vi "Magnetic Sweep 1.2.vi"() -> ()   [LabVIEW 2011]
uses:
  <vilib>/Math Plots/3D Math Plots/3D Contour/3D Contour XCtrl/3D Contour.xctl
  <vilib>/Math Plots/3D Math Plots/3D Contour/3D Contour Datatype/Public/Plot Helper (Vector).vi
  <vilib>/Math Plots/3D Math Plots/3D Contour/3D Contour Datatype/3D Contour Datatype.lvclass
panel:
  out "PID command":string
  out "setpoint command":string
  out "setpoint":dbl
  out "3D Contour \n(Ramp down)":refnum<class "3D Plot Datatype.lvclass">[](xcontrol)
  out "3D Contour\n(Ramp up)":refnum<class "3D Plot Datatype.lvclass">[](xcontrol)
  in  "stop":bool
  out "error out 3":errorcluster
  out "error out 2":errorcluster
  in  "Contour plot (ramp down)":path
  in  "Raw data (ramp down)":path
  out "Elapsed Time (s)":dbl
  out "Numeric":i32
  in  "error out":errorcluster
  out "Initial Temperature":string
  out "Zero field reached":bool
  out "Target field reached":bool
  in  "Upper limite":dbl
  in  "Temperature\nramping step":dbl
  in  "Heater range":i16(ring) items=["High", "Medium", "Low"]
  in  "D gain":dbl
  in  "I gain":dbl
  in  "P gain":dbl
  in  "Contour plot (ramp up)":path
  out "Time elapsed":string
  in  "Timer":bool caption="Reset"
  in  "date format":enum16{"short", "long", "abbreviated"}(ring)
  in  "Save":bool
  in  "Raw data (ramp  up)":path
  out "Temperature vs Time":cluster{dbl[], dbl[]}(graph)
  out "current time":timestamp
  out "Magnetic\nField":cluster{dbl[], dbl[]}(graph)
  out "Current Resistance":string
  out "Current Temperature":string
  out "Current Field":string
  out "Status":string
  in  "Field Sweep":bool
  in  "Start":bool
  out "Parameter\nSetup":string
  in  "Magnetic field\nRamp rate":dbl
  in  "Traget Field":dbl
  out "Init Response":string
  in  "error in (no error)":errorcluster
  in  "IP Address":string
  in  "Ramp":bool
  in  "Update":bool
  in  "Ramp to Zero":bool
  in  "P Switch":bool
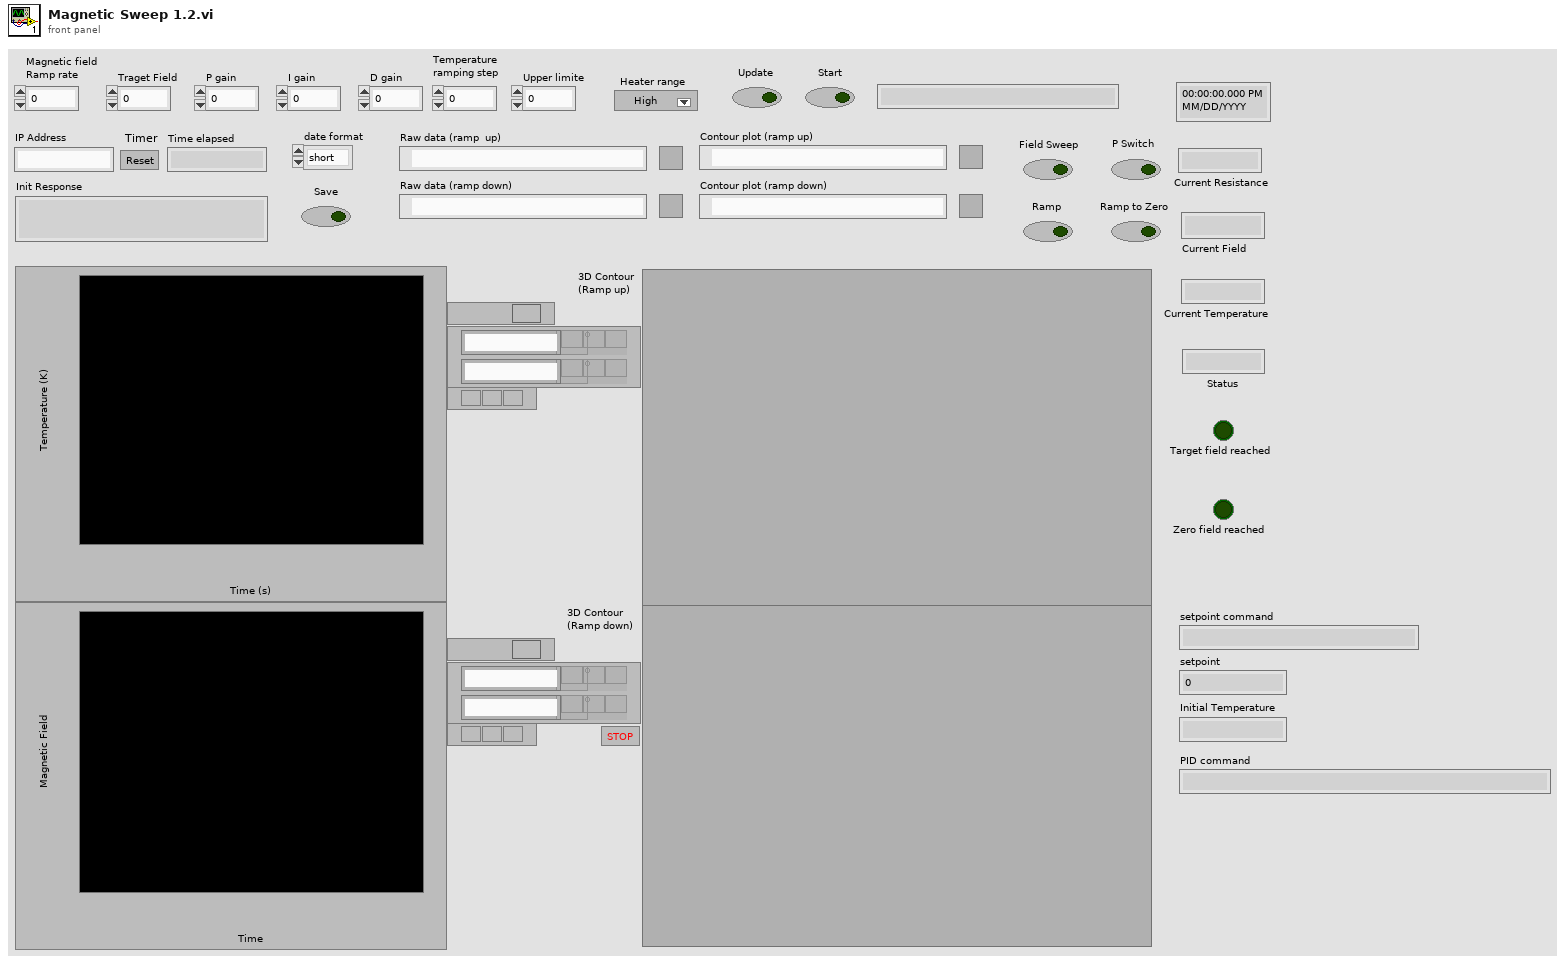
[diagram p1: front panel]
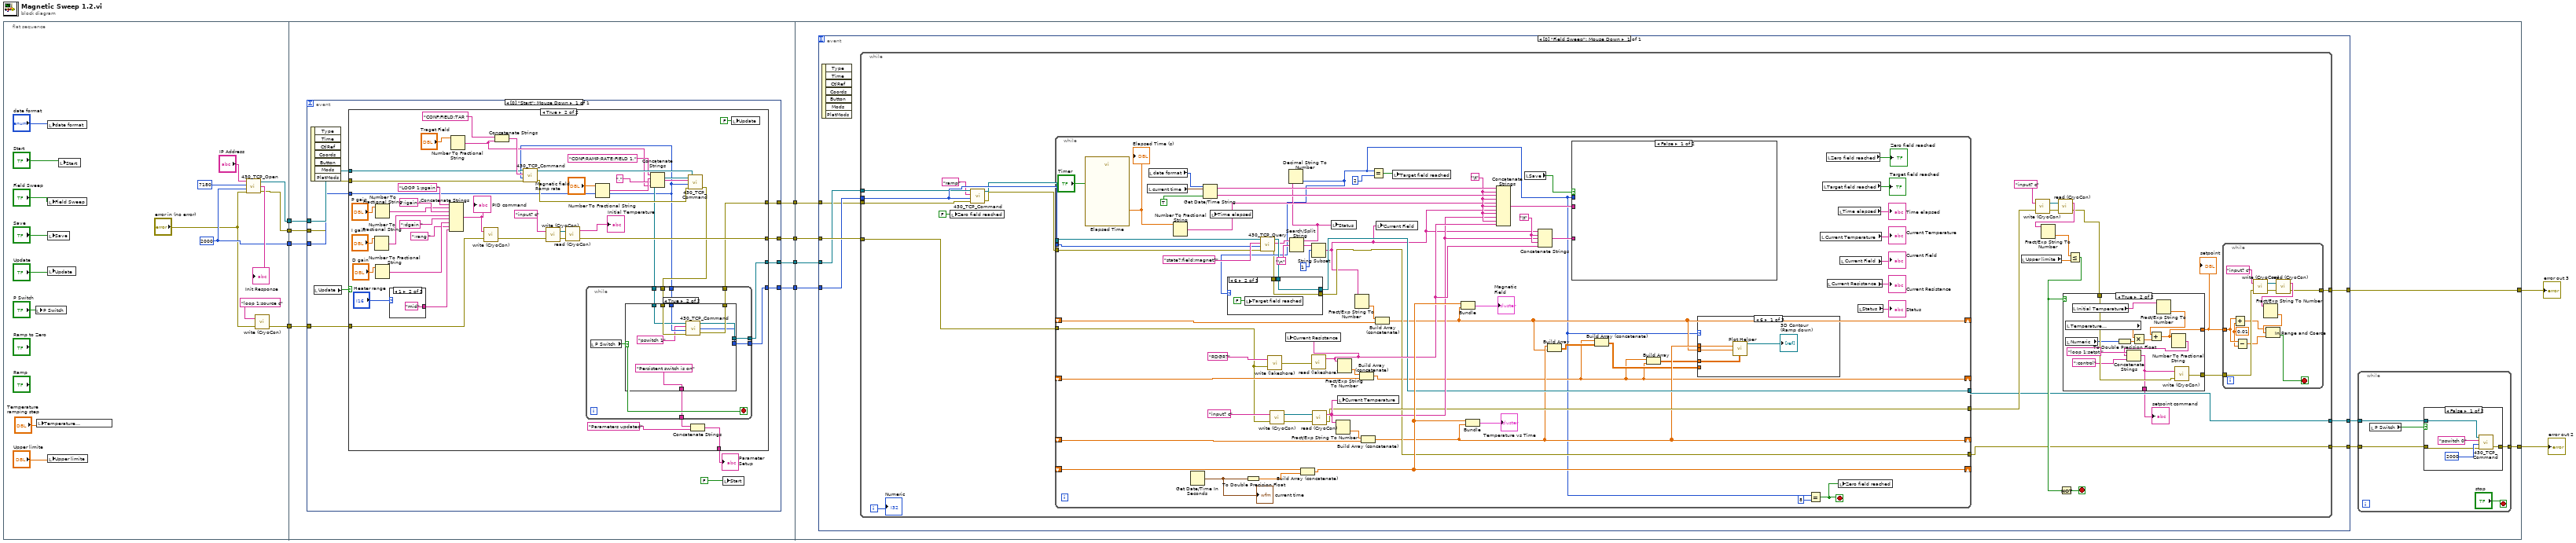
[diagram p0: block diagram]
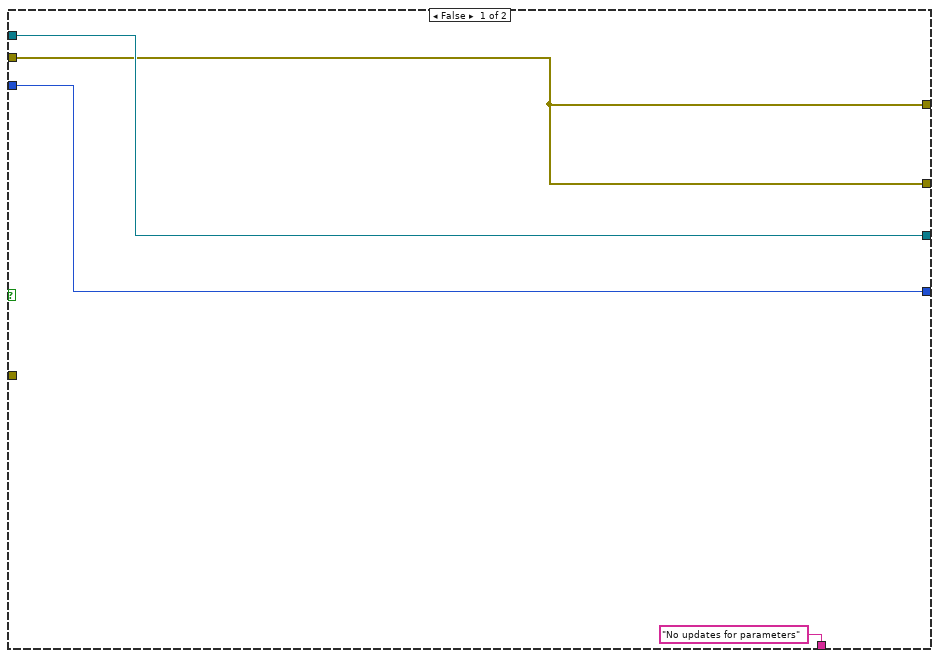
[diagram p2: hidden frame]
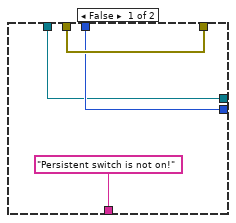
[diagram p3: hidden frame]
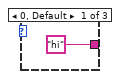
[diagram p4: hidden frame]
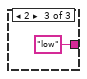
[diagram p5: hidden frame]
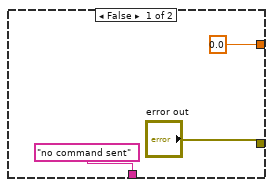
[diagram p7: hidden frame]
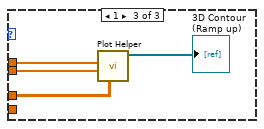
[diagram p9: hidden frame]
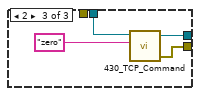
[diagram p11: hidden frame]
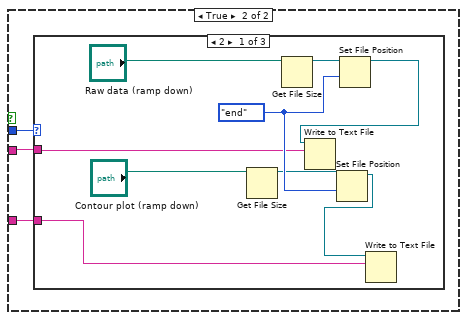
[diagram p12: hidden frame]
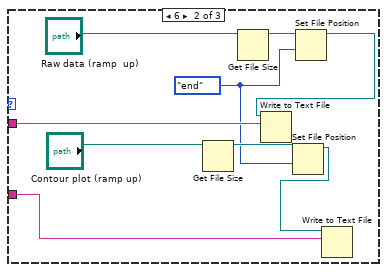
[diagram p13: hidden frame]
diagram:
  n1 = flat-sequence {
    tunnel: [w23] -> w10
    tunnel: [w22] -> w9
    tunnel: [w21] -> w8
    tunnel: [w17] -> w5
    tunnel: w10 -> [w35]
    tunnel: w9 -> [w34]
    tunnel: w8 -> [w33]
    tunnel: [w32] -> w7
    tunnel: [w31] -> w6
    tunnel: w5 -> [w30]
    tunnel: [w29] -> w4
    tunnel: [w28] -> w3
    tunnel: w7 -> [w124]
    tunnel: w6 -> [w123]
    tunnel: w4 -> [w122]
    tunnel: w3 -> [w121]
    tunnel: [w120] -> w2
    tunnel: [w118] -> w1
    frame #0 {
      w22 = 2000 ("Timeout")
      n2 = local write "P Switch"("P Switch") -> ()
      n3 = local write "Temperature\nramping step"("Temperature\nramping step") -> ()
      n4 = local write "date format"("date format") -> ()
      n5 = local write "Field Sweep"("Field Sweep") -> ()
      n6 = local write "Save"("Save") -> ()
      n7 = local write "Update"("Update") -> ()
      n8 = local write "Upper limite"("Upper limite") -> ()
      n9 = local write "Start"("Start") -> ()
      n10 = call "430_TCP_Open.vi"("IP Address"="IP Address", "TCP Port"=7180, "timeout ms (2000)"=w22, "error in (no error)"="error in (no error)") -> ("connection ID"=w23:refnum<k5>, "Init Response"=→"Init Response":string, "error out"=w21:errorcluster)  [unwired: 2 in]
      n11 = call "write (CryoCon).vi"("error in (no error)"="error in (no error)", "write buffer"="loop 1:source c") -> ("error out"=w17:errorcluster)  [unwired: 1 out]
    }
    frame #1 {
      n12 = event shown="[0] \"Start\": Mouse Down" {
        selector: _ -> [_]
        dyn-events: _ -> [_]
        timeout: _ -> [_]
        tunnel: w35 -> [w45]
        tunnel: w34 -> [w44]
        tunnel: w33 -> [w43]
        tunnel: [w42] -> w32
        tunnel: [w41] -> w31
        tunnel: w30 -> [w38]
        tunnel: [w37] -> w29
        tunnel: [w36] -> w28
        event "Start": Mouse Down {
          n13 = event-data() -> ()  [unwired: 1 in, 7 out]
          n14 = local read "Update"() -> (w46:bool)
          n15 = case shown="True" w46 {
            tunnel: w45 -> [w50 w91]
            tunnel: w44 -> [w49 w56]
            tunnel: w43 -> [w47 w80]
            tunnel: [w50 w55] -> w42
            tunnel: [w49 w54] -> w41
            tunnel: ["No updates for parameters" ("String") w51] -> w39
            tunnel: w38 -> [_ w69]
            tunnel: [w47 w61] -> w37
            tunnel: [w47 w58] -> w36
            frame False {
            }
            frame True {
              n16 = Number To Fractional String(number="I gain") -> (F-format string=w73:string)  [unwired: 3 in]
              n17 = Number To Fractional String(number="D gain") -> (F-format string=w71:string)  [unwired: 3 in]
              n18 = Number To Fractional String(number="P gain") -> (F-format string=w74:string)  [unwired: 3 in]
              n19 = case shown="1" "Heater range" {
                tunnel: ["hi" "mid" "low"] -> w66
                frame 0, Default {
                }
                frame 1 {
                }
                frame 2 {
                }
              }
              n20 = Concatenate Strings("LOOP 1:pgain " ("write buffer"), w74, ";igain " ("string"), w73, ";dgain " ("string"), w71, ";rang " ("string"), w66) -> (w70:string)
              "PID command" <- w70
              n21 = Number To Fractional String(number="Traget Field") -> (F-format string=w81:string)  [unwired: 3 in]
              n22 = call "write (CryoCon).vi"("error in (no error)"=w69, "write buffer"=w70) -> ("error out"=w62:errorcluster)  [unwired: 1 out]
              n23 = Concatenate Strings("CONF:FIELD:TAR ", w81) -> (w92:string)
              n24 = call "430_TCP_Command.vi"("error in (no error)"=w80, "Timeout"=w56, "Command"=w92, "connection ID"=w91) -> ("error out"=w90:errorcluster, "connection ID out"=w86:refnum<k5>)  [unwired: 1 out]
              n25 = call "write (CryoCon).vi"("error in (no error)"=w62, "write buffer"="input? c") -> ("error out"=w65:errorcluster, "VISA resource name out"=w64:refnum<visa-resource-name>)
              n26 = call "read (CryoCon).vi"("error in (no error)"=w65, "VISA resource name"=w64) -> ("error out"=w61:errorcluster, "read buffer"=→"Initial Temperature":string)
              n27 = Number To Fractional String(number="Magnetic field\nRamp rate") -> (F-format string=w84:string)  [unwired: 3 in]
              n28 = Concatenate Strings("CONF:RAMP:RATE:FIELD 1," ("string"), w84, "," ("string"), w81) -> (w87:string)
              n29 = call "430_TCP_Command.vi"("error in (no error)"=w90, "Timeout"=w56, "Command"=w87, "connection ID"=w86) -> ("error out"=w59:errorcluster, "connection ID out"=w57:refnum<k5>)  [unwired: 1 out]
              n30 = while {
                tunnel: w59 -> [w101]
                tunnel: [w100] -> w58
                tunnel: w57 -> [w99]
                tunnel: w56 -> [w98]
                tunnel: [w97] -> w55
                tunnel: [w96] -> w54
                tunnel: [w94] -> w52
                stop <- w95 stop-if-true
                n31 = local read "P Switch"() -> (w95:bool)
                n32 = case shown="True" w95 {
                  tunnel: w101 -> [w105 w113]
                  tunnel: [w105 w112] -> w100
                  tunnel: w99 -> [w103 w111]
                  tunnel: w98 -> [w104 w110]
                  tunnel: [w103 w109] -> w97
                  tunnel: [w104 w108] -> w96
                  tunnel: ["Persistent switch is not on!" "Persistent switch is on"] -> w94
                  frame False {
                  }
                  frame True {
                    n33 = call "430_TCP_Command.vi"("error in (no error)"=w113, "Timeout"=w110, "Command"="pswitch 1", "connection ID"=w111) -> ("error out"=w112:errorcluster, "bytes written"=w108:i32, "connection ID out"=w109:refnum<k5>)
                  }
                }
              }
              n34 = Concatenate Strings(w52, "Parameters updated" ("String")) -> (w51:string)
              n35 = local write "Update"(FALSE ("Update")) -> ()
            }
          }
          "Parameter\nSetup" <- w39
          n36 = local write "Start"(FALSE ("Set Parameter")) -> ()
        }
      }
    }
    frame #2 {
      n37 = event shown="[0] \"Field Sweep\": Mouse Down" {
        selector: _ -> [_]
        dyn-events: _ -> [_]
        timeout: _ -> [_]
        tunnel: w124 -> [w141]
        tunnel: w123 -> [w140]
        tunnel: w122 -> [w142]
        tunnel: w121 -> [w139]
        tunnel: [w138] -> w120
        tunnel: [w137] -> w119
        tunnel: [w136] -> w117
        event "Field Sweep": Mouse Down {
          n38 = event-data() -> ()  [unwired: 1 in, 7 out]
          n39 = while {
            tunnel: w142 -> [w162]
            tunnel: w140 -> [w166]
            tunnel: w141 -> [w165]
            tunnel: w139 -> [w163]
            tunnel: [w146] -> w138
            tunnel: [w145] -> w137
            tunnel: [w144] -> w136
            i -> [w159]
            stop <- w148 stop-if-true
            n40 = local write "Zero field reached"(FALSE ("Zero field reached")) -> ()
            n41 = call "430_TCP_Command.vi"("error in (no error)"=w163, "Timeout"=w166, "Command"="ramp", "connection ID"=w165) -> ("error out"=w167:errorcluster, "connection ID out"=w164:refnum<k5>)  [unwired: 1 out]
            n42 = while {
              shift-right: [w201] -> _
              shift-left: _ -> [w252]
              shift-right: [w202] -> _
              shift-left: _ -> [w257]
              shift-right: [w198] -> _
              shift-left: _ -> [w254]
              shift-right: [w247] -> _
              shift-left: _ -> [w248]
              tunnel: w167 -> [w236]
              tunnel: w166 -> [w213]
              tunnel: w164 -> [w235]
              tunnel: w162 -> [w229]
              tunnel: [w223] -> w149
              tunnel: [w211] -> w145
              tunnel: [w210] -> w144
              stop <- w215 stop-if-true
              w240 = "\t"
              w241 = "\t"
              n43 = call "Elapsed Time"("Reset"="Timer") -> ("Elapsed Time (s)"=w227:dbl)  [unwired: 11 in, 7 out]
              "Elapsed Time (s)" <- w227
              n44 = local read "current time"() -> (w238:timestamp)
              n45 = local read "date format"() -> (w230:enum16{"short", "long", "abbreviated"})
              n46 = Number To Fractional String(number=w227) -> (F-format string=w233:string)  [unwired: 3 in]
              n47 = Get Date/Time In Seconds() -> (seconds since 1Jan1904=w226:timestamp)
              "current time" <- w226
              n48 = Get Date/Time String(date format (0)=w230, seconds (now)=w238, want seconds? (F)=TRUE) -> (date string=w243:string, time string=w242:string)
              n49 = local write "Time elapsed"(w233) -> ()
              n50 = To Double Precision Float(number=w226) -> (double precision float=w249:dbl)
              n51 = call "430_TCP_Query.vi"("error in (no error)"=w236, "Timeout"=w213, "Command"="state?;field:magnet?", "connection ID"=w235) -> ("error out"=w196:errorcluster, "Response"=w209:string, "connection ID out"=w214:refnum<k5>)  [unwired: 3 in, 2 out]
              n52 = call "write (lakeshore).vi"("error in (no error)"=w229, "write buffer"="RDGR?") -> ("error out"=w256:errorcluster)
              n53 = call "write (CryoCon).vi"("error in (no error)"=w229, "write buffer"="input? c") -> ("error out"=w258:errorcluster, "VISA resource name out"=w259:refnum<visa-resource-name>)
              n54 = Search/Split String(string=w209, search string/char (-)="\n") -> (substring before match=w208:string, match + rest of string=w207:string)  [unwired: 1 in, 1 out]
              n55 = Decimal String To Number(string=w208) -> (number=w197:i32)  [unwired: 2 in, 1 out]
              n56 = case shown="6" w197 {
                tunnel: [w270 w272 w277] -> w210
                tunnel: w214 -> [w271 w274 w276]
                tunnel: [w271 w274 w275] -> w211
                tunnel: w196 -> [w270 w272 _]
                frame 0, Default {
                }
                frame 6 {
                  n57 = local write "Target field reached"(FALSE ("Target field reached")) -> ()
                }
                frame 2 {
                  n58 = call "430_TCP_Command.vi"("Command"="zero", "connection ID"=w276) -> ("error out"=w277:errorcluster, "connection ID out"=w275:refnum<k5>)  [unwired: 2 in, 1 out]
                }
              }
              n59 = Build Array (concatenate)(w248, w249) -> (w247:dbl[])
              n60 = call "read (lakeshore).vi"("error in (no error)"=w256) -> ("read buffer"=w232:string)  [unwired: 1 out]
              n61 = local write "Current Resistance"(w232) -> ()
              n62 = String Subset(string=w207, offset (0)=1) -> (substring=w205:string)  [unwired: 1 in]
              n63 = call "read (CryoCon).vi"("error in (no error)"=w258, "VISA resource name"=w259) -> ("error out"=w223:errorcluster, "read buffer"=w231:string)
              n64 = local write "Status"(w208) -> ()
              n65 = Fract/Exp String To Number(string=w231) -> (number=w251:dbl)  [unwired: 3 in, 1 out]
              n66 = Fract/Exp String To Number(string=w232) -> (number=w250:dbl)  [unwired: 3 in, 1 out]
              n67 = local write "Current Temperature"(w231) -> ()
              n68 = Fract/Exp String To Number(string=w205) -> (number=w253:dbl)  [unwired: 3 in, 1 out]
              n69 = Build Array (concatenate)(w250, w254) -> (w198:dbl[])
              n70 = Build Array (concatenate)(w251, w257) -> (w202:dbl[])
              n71 = Equal?(x=w197, y=2) -> (x = y?=w234:bool)
              n72 = Build Array (concatenate)(w253, w252) -> (w201:dbl[])
              n73 = local write "Current Field"(w205) -> ()
              n74 = local write "Target field reached"(w234) -> ()
              n75 = Bundle(w247, w201) -> (→"Magnetic\nField":cluster{dbl[], dbl[]})  [unwired: 1 in]
              n76 = Bundle(w247, w202) -> (→"Temperature vs Time":cluster{dbl[], dbl[]})  [unwired: 1 in]
              n77 = Concatenate Strings(w243, w241, w242, w241, w233, w241, w205, w241, w231, w241, w232) -> (w246:string)
              n78 = local read "Save"() -> (w225:bool)
              n79 = Concatenate Strings(w205, w240, w231, w240, w232) -> (w239:string)
              n80 = Build Array(w202, w201) -> (w212:dbl[][])
              n81 = case shown="False" w225 {
                tunnel: w246 -> [_ w281]
                tunnel: w239 -> [_ w280]
                tunnel: w197 -> [_ w279]
                frame False {
                }
                frame True {
                  n82 = case shown="2" w279 {
                    tunnel: w281 -> [w283 w299 _]
                    tunnel: w280 -> [w282 w293 _]
                    frame 2 {
                      w289 = enum16{"start", "end", "current"}."end" ("from (0:start)")
                      n83 = Get File Size(file="Contour plot (ramp down)") -> (refnum out=w288:refnum<file>)  [unwired: 1 in, 2 out]
                      n84 = Get File Size(file="Raw data (ramp down)") -> (refnum out=w285:refnum<file>)  [unwired: 1 in, 2 out]
                      n85 = Set File Position(refnum=w288, from (0:start)=w289) -> (refnum out=w290:refnum<file>)  [unwired: 2 in, 1 out]
                      n86 = Set File Position(refnum=w285, from (0:start)=w289) -> (refnum out=w286:refnum<file>)  [unwired: 2 in, 1 out]
                      n87 = Write to Text File(file (use dialog)=w286, text=w283) -> ()  [unwired: 2 in, 3 out]
                      n88 = Write to Text File(file (use dialog)=w290, text=w282) -> ()  [unwired: 2 in, 3 out]
                    }
                    frame 6 {
                      w292 = enum16{"start", "end", "current"}."end" ("from (0:start)")
                      n89 = Get File Size(file="Contour plot (ramp up)") -> (refnum out=w294:refnum<file>)  [unwired: 1 in, 2 out]
                      n90 = Get File Size(file="Raw data (ramp  up)") -> (refnum out=w297:refnum<file>)  [unwired: 1 in, 2 out]
                      n91 = Set File Position(refnum=w294, from (0:start)=w292) -> (refnum out=w291:refnum<file>)  [unwired: 2 in, 1 out]
                      n92 = Set File Position(refnum=w297, from (0:start)=w292) -> (refnum out=w296:refnum<file>)  [unwired: 2 in, 1 out]
                      n93 = Write to Text File(file (use dialog)=w296, text=w299) -> ()  [unwired: 2 in, 3 out]
                      n94 = Write to Text File(file (use dialog)=w291, text=w293) -> ()  [unwired: 2 in, 3 out]
                    }
                    frame Default {
                    }
                  }
                }
              }
              n95 = Build Array (concatenate)(w198, w212) -> (w199:dbl[][])
              n96 = Build Array(w198, w198) -> (w200:dbl[][])
              n97 = case shown="6" w197 {
                tunnel: w202 -> [w264 _ w268]
                tunnel: w201 -> [w263 _ w267]
                tunnel: w200 -> [w262 _ w266]
                tunnel: w199 -> [_ _ _]
                frame 6 {
                  n98 = call-poly <vilib>:"Plot Helper.vi"("z matrix"=w262, "y vector"=w263, "x vector"=w264) -> ("3D Plot lvclass Array out"=→"3D Contour \n(Ramp down)":refnum<class "3D Plot Datatype.lvclass">[])  [unwired: 3 in, 5 out]
                }
                frame 0, Default {
                }
                frame 1 {
                  n99 = call-poly <vilib>:"Plot Helper.vi"("z matrix"=w266, "y vector"=w267, "x vector"=w268) -> ("3D Plot lvclass Array out"=→"3D Contour\n(Ramp up)":refnum<class "3D Plot Datatype.lvclass">[])  [unwired: 3 in, 5 out]
                }
              }
              n100 = Equal?(x=w197, y=8) -> (x = y?=w215:bool)
              n101 = local read "Current Temperature"() -> (→"Current Temperature":string)
              n102 = local read "Target field reached"() -> (→"Target field reached":bool)
              n103 = local read "Zero field reached"() -> (→"Zero field reached":bool)
              n104 = local read "Current Resistance"() -> (→"Current Resistance":string)
              n105 = local read "Time elapsed"() -> (→"Time elapsed":string)
              n106 = local write "Zero field reached"(w215) -> ()
              n107 = local read "Current Field"() -> (→"Current Field":string)
              n108 = local read "Status"() -> (→"Status":string)
            }
            n109 = local read "Upper limite"() -> (w151:dbl)
            n110 = call "write (CryoCon).vi"("error in (no error)"=w149, "write buffer"="input? c") -> ("error out"=w154:errorcluster, "VISA resource name out"=w155:refnum<visa-resource-name>)
            n111 = call "read (CryoCon).vi"("error in (no error)"=w154, "VISA resource name"=w155) -> ("error out"=w152:errorcluster, "read buffer"=w153:string)
            n112 = Fract/Exp String To Number(string=w153) -> (number=w150:dbl)  [unwired: 3 in, 1 out]
            n113 = Less Or Equal?(x=w150, y=w151) -> (x <= y?=w147:bool)
            n114 = Not(x=w147) -> (.not. x?=w148:bool)
            n115 = case shown="True" w147 {
              tunnel: w152 -> [_ w193]
              tunnel: ["error out" w190] -> w161
              tunnel: [0.0 w189] -> w160
              tunnel: ["no command sent" w183] -> w143
              frame False {
              }
              frame True {
                n116 = local read "Temperature\nramping step"() -> (w187:dbl)
                n117 = local read "Numeric"() -> (w185:i32)
                n118 = local read "Initial Temperature"() -> (w192:string)
                n119 = To Double Precision Float(number=w185) -> (double precision float=w186:dbl)
                n120 = Multiply(x=w187, y=w186) -> (x*y=w188:dbl)
                n121 = Fract/Exp String To Number(string=w192) -> (number=w191:dbl)  [unwired: 3 in, 1 out]
                n122 = Add(x=w191, y=w188) -> (x+y=w189:dbl)
                n123 = Number To Fractional String(number=w189) -> (F-format string=w194:string)  [unwired: 3 in]
                n124 = Concatenate Strings("loop 1:setpt " ("write buffer"), w194, ";control" ("string")) -> (w183:string)
                n125 = call "write (CryoCon).vi"("error in (no error)"=w193, "write buffer"=w183) -> ("error out"=w190:errorcluster)  [unwired: 1 out]
              }
            }
            "setpoint" <- w160
            "setpoint command" <- w143
            n126 = while {
              tunnel: w161 -> [w178]
              tunnel: w160 -> [w173]
              tunnel: [w168] -> w146
              stop <- w169 stop-if-true
              w170 = 0.01 ("y")
              n127 = Add(x=w173, y=w170) -> (x+y=w172:dbl)
              n128 = Subtract(x=w173, y=w170) -> (x-y=w171:dbl)
              n129 = call "write (CryoCon).vi"("error in (no error)"=w178, "write buffer"="input? c") -> ("error out"=w177:errorcluster, "VISA resource name out"=w179:refnum<visa-resource-name>)
              n130 = call "read (CryoCon).vi"("error in (no error)"=w177, "VISA resource name"=w179) -> ("error out"=w168:errorcluster, "read buffer"=w175:string)
              n131 = Fract/Exp String To Number(string=w175) -> (number=w174:dbl)  [unwired: 3 in, 1 out]
              n132 = In Range and Coerce(upper limit=w172, x=w174, lower limit=w171) -> (In Range?=w169:bool)  [unwired: 1 out]
            }
            "Numeric" <- w159
          }
        }
      }
      n133 = while {
        tunnel: w119 -> [w129]
        tunnel: [w127] -> w118
        tunnel: w117 -> [w126]
        stop <- "stop" stop-if-true
        n134 = local read "P Switch"() -> (w128:bool)
        n135 = case shown="False" w128 {
          tunnel: w129 -> [w133 _]
          tunnel: [w131 w135] -> w127
          tunnel: w126 -> [w130 w135]
          frame False {
            n136 = call "430_TCP_Command.vi"("error in (no error)"=w130, "Timeout"=2000, "Command"="pswitch 0", "connection ID"=w133) -> ("error out"=w131:errorcluster)  [unwired: 2 out]
          }
          frame True {
          }
        }
      }
    }
  }
  "error out 2" <- w1
  "error out 3" <- w2
